vi "Run_Wavedump.vi"(6 "Close":bool, 7 "Start":bool, 8 "Channel":string[](array[string]), 9 "PMTs":string[](array[string]), 11 "Test":string(combo)) -> (0 "Error":string="\n", 1 "Event Build Error":bool, 2 "Over Temperature":bool, 3 "Command Line Output":string)   [LabVIEW 2018]
panel:
  in  "Tab Control":enum32{"Controls", "Read Me"}(tab)
  out "Files Moved":bool
  out "Bash Script Run":bool=TRUE
  in  "View PMT Files":bool
  in  "Run":string
  in  "Time":string
  # "This application is used to send a command to run the bash script relating to an electrical test for PMTs.\n\nThe bash script will run wavedump in a preset configuration.\n\nUse the Controls tab to send the necessary commands.\n\nTo run, enter up to 8 PMT numbers and the channels they are connected to on the digitiser.\n\nSelect the test to run and press \"Start\".\n\nA window will pop up to display the waveform as it is being recorded.\n\nTo view other PMT files or scroll through the ones being recorded, press \"View PMT Files\".\n\nAs the program only sends a command, it can't be used to stop or control wavedump.\n\nPress \"CLOSE\" to close the application."
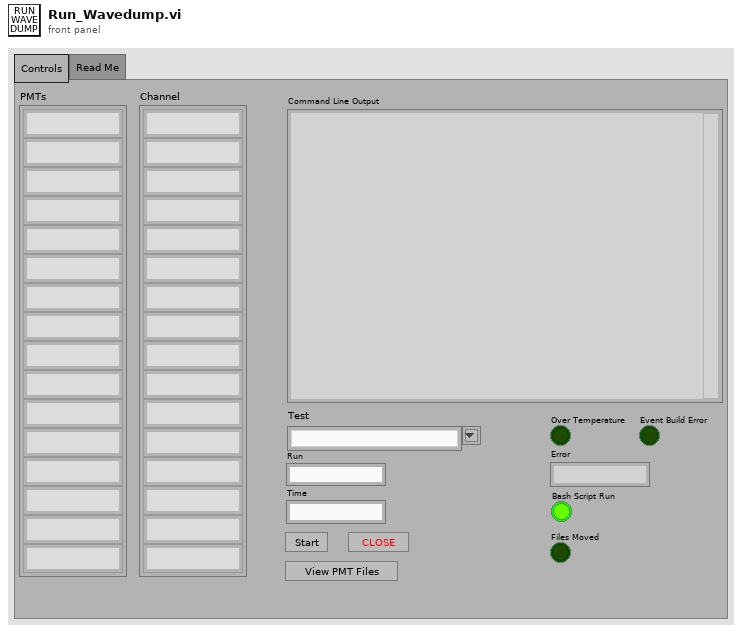
[diagram p1: front panel]
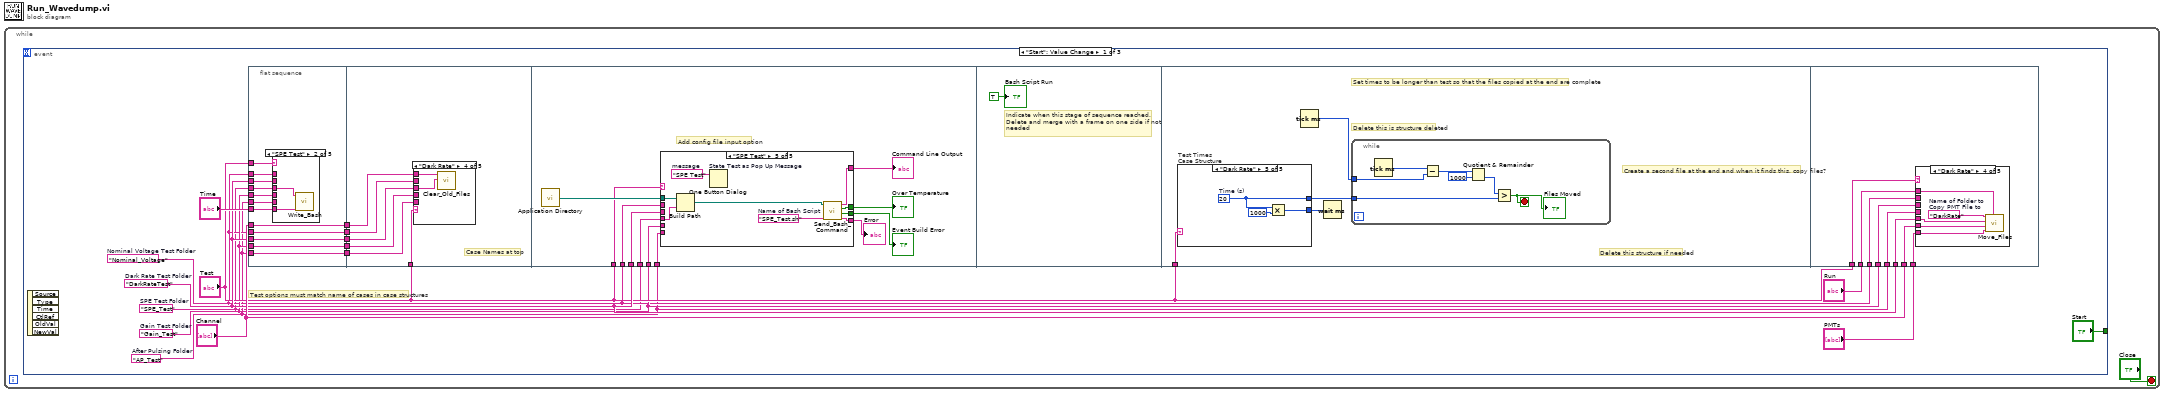
[diagram p0: block diagram]
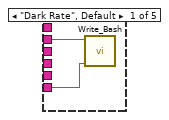
[diagram p2: hidden frame]
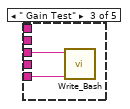
[diagram p3: hidden frame]
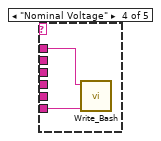
[diagram p4: hidden frame]
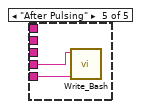
[diagram p5: hidden frame]
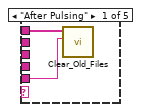
[diagram p6: hidden frame]
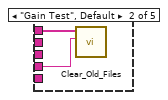
[diagram p7: hidden frame]
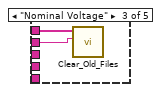
[diagram p8: hidden frame]
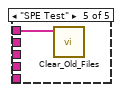
[diagram p9: hidden frame]
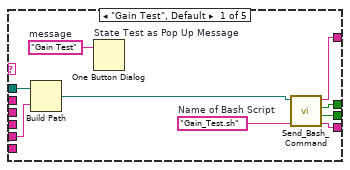
[diagram p10: hidden frame]
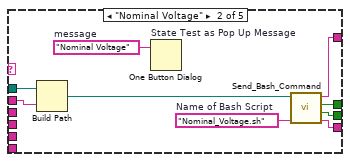
[diagram p11: hidden frame]
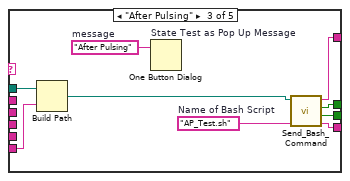
[diagram p12: hidden frame]
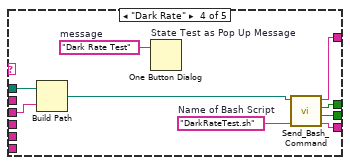
[diagram p13: hidden frame]
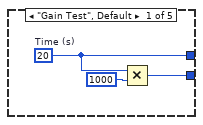
[diagram p14: hidden frame]
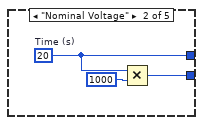
[diagram p15: hidden frame]
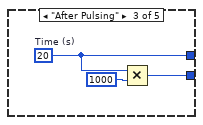
[diagram p16: hidden frame]
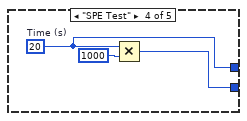
[diagram p17: hidden frame]
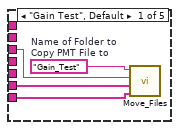
[diagram p18: hidden frame]
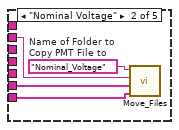
[diagram p19: hidden frame]
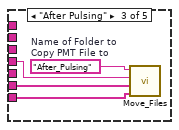
[diagram p20: hidden frame]
diagram:
  n1 = while {
    stop <- "Close" stop-if-true
    n2 = event shown="[0] \"Start\": Value Change" {
      selector: _ -> [_ _ _]
      dyn-events: _ -> [_ _ _]
      timeout: _ -> [_ _ _]
      tunnel: ["Start" "View PMT Files" w170] -> _
      event "Start": Value Change {
        w2 = "SPE_Test"  # SPE Test Folder
        w3 = "AP_Test"  # After Pulsing Folder
        w7 = "DarkRateTest"  # Dark Rate Test Folder
        w4 = "Nominal_Voltage"  # Nominal Voltage Test Folder
        w5 = "Gain_Test"  # Gain Test Folder
        # "Test options must match name of cases in case structures"
        n3 = event-data() -> ()  [unwired: 1 in, 6 out]
        n4 = flat-sequence {
          tunnel: w5 -> [w25]
          tunnel: w3 -> [w26]
          tunnel: w7 -> [w27]
          tunnel: w4 -> [w28]
          tunnel: "Channel" -> [w29]
          tunnel: [w29] -> w13
          tunnel: [w28] -> w12
          tunnel: [w27] -> w11
          tunnel: [w26] -> w10
          tunnel: [w25] -> w9
          tunnel: "Test" -> [w24]
          tunnel: "Time" -> [w23]
          tunnel: w7 -> [w22]
          tunnel: w5 -> [w21]
          tunnel: w4 -> [w20]
          tunnel: w3 -> [w19]
          tunnel: w2 -> [w18]
          tunnel: w13 -> [w45]
          tunnel: w12 -> [w44]
          tunnel: w11 -> [w43]
          tunnel: w10 -> [w42]
          tunnel: w9 -> [w41]
          tunnel: "Test" -> [w40]
          tunnel: "Test" -> [w60]
          tunnel: w5 -> [w59]
          tunnel: w4 -> [w58]
          tunnel: w7 -> [w57]
          tunnel: w3 -> [w56]
          tunnel: w2 -> [w55]
          tunnel: "Test" -> [w114]
          tunnel: "PMTs" -> [w142]
          tunnel: "Test" -> [w145]
          tunnel: w3 -> [w144]
          tunnel: "Channel" -> [w143]
          tunnel: w7 -> [w141]
          tunnel: w5 -> [w140]
          tunnel: w4 -> [w139]
          tunnel: "Run" -> [w138]
          frame #0 {
            n5 = case shown="\"SPE Test\"" w24 {
              tunnel: w23 -> [w31 w33 w34 w36 w38]
              tunnel: w22 -> [w30 _ _ _ _]
              tunnel: w21 -> [_ _ w35 _ _]
              tunnel: w20 -> [_ _ _ w37 _]
              tunnel: w19 -> [_ _ _ _ w39]
              tunnel: w18 -> [_ w32 _ _ _]
              frame "Dark Rate", Default {
                n6 = call "Write_Bash.vi"("Time"=w31, "Test"=w30) -> ()  [unwired: 10 in]
              }
              frame "SPE Test" {
                n7 = call "Write_Bash.vi"("Time"=w33, "Test"=w32) -> ()  [unwired: 10 in]
              }
              frame " Gain Test" {
                n8 = call "Write_Bash.vi"("Time"=w34, "Test"=w35) -> ()  [unwired: 10 in]
              }
              frame "Nominal Voltage" {
                n9 = call "Write_Bash.vi"("Time"=w36, "Test"=w37) -> ()  [unwired: 10 in]
              }
              frame "After Pulsing" {
                n10 = call "Write_Bash.vi"("Time"=w38, "Test"=w39) -> ()  [unwired: 10 in]
              }
            }
          }
          frame #1 {
            # "Case Names at top"
            n11 = case shown="\"Dark Rate\"" w40 {
              tunnel: w45 -> [w47 w49 w51 w53 w54]
              tunnel: w44 -> [_ _ w50 _ _]
              tunnel: w43 -> [_ _ _ w52 _]
              tunnel: w42 -> [w46 _ _ _ _]
              tunnel: w41 -> [_ w48 _ _ _]
              frame "After Pulsing" {
                n12 = call "Clear_Old_Files.vi"("Bash Script Folder Name"=w46, "Channel"=w47) -> ()  [unwired: 10 in]
              }
              frame "Gain Test", Default {
                n13 = call "Clear_Old_Files.vi"("Bash Script Folder Name"=w48, "Channel"=w49) -> ()  [unwired: 10 in]
              }
              frame "Nominal Voltage" {
                n14 = call "Clear_Old_Files.vi"("Bash Script Folder Name"=w50, "Channel"=w51) -> ()  [unwired: 10 in]
              }
              frame "Dark Rate" {
                n15 = call "Clear_Old_Files.vi"("Bash Script Folder Name"=w52, "Channel"=w53) -> ()  [unwired: 10 in]
              }
              frame "SPE Test" {
                n16 = call "Clear_Old_Files.vi"("Channel"=w54) -> ()  [unwired: 11 in]
              }
            }
          }
          frame #2 {
            # "Add config file input option"
            n17 = call <vilib>:"Application Directory.vi"() -> ("Application Directory"=w65:path)
            n18 = case shown="\"SPE Test\"" w60 {
              tunnel: [w66 w75 w84 w93 w103] -> w61
              tunnel: [w67 w76 w85 w94 w104] -> w62
              tunnel: [w68 w77 w86 w95 w105] -> w63
              tunnel: [w69 w78 w87 w96 w106] -> w64
              tunnel: w65 -> [w71 w80 w88 w99 w107]
              tunnel: w59 -> [w70 _ _ _ _]
              tunnel: w58 -> [_ w79 _ _ _]
              tunnel: w57 -> [_ _ _ w97 _]
              tunnel: w56 -> [_ _ w89 _ _]
              tunnel: w55 -> [_ _ _ _ w102]
              frame "Gain Test", Default {
                w73 = "Gain Test"  # message
                w74 = "Gain_Test.sh"  # Name of Bash Script
                n19 = Build Path(base path=w71, name or relative path=w70) -> (appended path=w72:path)
                n20 = One Button Dialog "State Test as Pop Up Message"(message=w73) -> ()  [unwired: 1 in, 1 out]
                n21 = call "Send_Bash_Command.vi"("working directory"=w72, "Bash script"=w74) -> ("Command Line Output"=w69:string, "Over Temperature"=w68:bool, "Event Build Error"=w67:bool, "Error"=w66:string)  [unwired: 5 in]
              }
              frame "Nominal Voltage" {
                w82 = "Nominal Voltage"  # message
                w83 = "Nominal_Voltage.sh"  # Name of Bash Script
                n22 = Build Path(base path=w80, name or relative path=w79) -> (appended path=w81:path)
                n23 = One Button Dialog "State Test as Pop Up Message"(message=w82) -> ()  [unwired: 1 in, 1 out]
                n24 = call "Send_Bash_Command.vi"("working directory"=w81, "Bash script"=w83) -> ("Command Line Output"=w78:string, "Over Temperature"=w77:bool, "Event Build Error"=w76:bool, "Error"=w75:string)  [unwired: 5 in]
              }
              frame "After Pulsing" {
                w91 = "After Pulsing"  # message
                w92 = "AP_Test.sh"  # Name of Bash Script
                n25 = Build Path(base path=w88, name or relative path=w89) -> (appended path=w90:path)
                n26 = One Button Dialog "State Test as Pop Up Message"(message=w91) -> ()  [unwired: 1 in, 1 out]
                n27 = call "Send_Bash_Command.vi"("working directory"=w90, "Bash script"=w92) -> ("Command Line Output"=w87:string, "Over Temperature"=w86:bool, "Event Build Error"=w85:bool, "Error"=w84:string)  [unwired: 5 in]
              }
              frame "Dark Rate" {
                w101 = "Dark Rate Test"  # message
                w98 = "DarkRateTest.sh"  # Name of Bash Script
                n28 = Build Path(base path=w99, name or relative path=w97) -> (appended path=w100:path)
                n29 = One Button Dialog "State Test as Pop Up Message"(message=w101) -> ()  [unwired: 1 in, 1 out]
                n30 = call "Send_Bash_Command.vi"("working directory"=w100, "Bash script"=w98) -> ("Command Line Output"=w96:string, "Over Temperature"=w95:bool, "Event Build Error"=w94:bool, "Error"=w93:string)  [unwired: 5 in]
              }
              frame "SPE Test" {
                w109 = "SPE Test"  # message
                w110 = "SPE_Test.sh"  # Name of Bash Script
                n31 = Build Path(base path=w107, name or relative path=w102) -> (appended path=w108:path)
                n32 = One Button Dialog "State Test as Pop Up Message"(message=w109) -> ()  [unwired: 1 in, 1 out]
                n33 = call "Send_Bash_Command.vi"("working directory"=w108, "Bash script"=w110) -> ("Command Line Output"=w106:string, "Over Temperature"=w105:bool, "Event Build Error"=w104:bool, "Error"=w103:string)  [unwired: 5 in]
              }
            }
            "Command Line Output" <- w64
            "Over Temperature" <- w63
            "Event Build Error" <- w62
            "Error" <- w61
          }
          frame #3 {
            # "Indicate when this stage of sequence reached.\nDelete and merge with a frame on one side if not needed"
            "Bash Script Run" <- TRUE
          }
          frame #4 {
            # "Create a second file at the end and when it finds this, copy files?"
            # "Delete this is structure deleted"
            # "Delete this structure if needed"
            # "Set times to be longer than test so that the files copied at the end are complete"
            n34 = case "Test Times\nCase Structure" shown="\"Dark Rate\"" w114 {
              tunnel: [w124 w127 w130 w133 w137] -> w115
              tunnel: [w123 w126 w129 w132 w135] -> w112
              frame "Gain Test", Default {
                w123 = u32 20  # Time (s)
                n35 = Multiply(x=w123, y=u32 1000) -> (x*y=w124:u32)
              }
              frame "Nominal Voltage" {
                w126 = u32 20  # Time (s)
                n36 = Multiply(x=w126, y=u32 1000) -> (x*y=w127:u32)
              }
              frame "After Pulsing" {
                w129 = u32 20  # Time (s)
                n37 = Multiply(x=w129, y=u32 1000) -> (x*y=w130:u32)
              }
              frame "SPE Test" {
                w132 = u32 20  # Time (s)
                n38 = Multiply(x=w132, y=u32 1000) -> (x*y=w133:u32)
              }
              frame "Dark Rate" {
                w135 = u32 20  # Time (s)
                n39 = Multiply(x=w135, y=u32 1000) -> (x*y=w137:u32)
              }
            }
            n40 = Tick Count (ms)() -> (millisecond timer value=w113:u32)
            n41 = Wait (ms)(milliseconds to wait=w115) -> ()  [unwired: 1 out]
            n42 = while {
              tunnel: w113 -> [w121]
              tunnel: w112 -> [w117]
              stop <- w116 stop-if-true
              n43 = Tick Count (ms)() -> (millisecond timer value=w122:u32)
              n44 = Subtract(x=w122, y=w121) -> (x-y=w120:u32)
              n45 = Quotient & Remainder(x=w120, y=u32 1000) -> (floor(x/y)=w118:u32)  [unwired: 1 out]
              n46 = Greater?(x=w118, y=w117) -> (0:w116:bool)
              "Files Moved" <- w116
            }
          }
          frame #5 {
            n47 = case shown="\"Dark Rate\"" w145 {
              tunnel: w144 -> [_ _ w157 _ _]
              tunnel: w143 -> [w147 w151 w155 w160 w164]
              tunnel: w142 -> [w146 w150 w154 w159 w163]
              tunnel: w141 -> [_ _ _ w161 _]
              tunnel: w140 -> [w148 _ _ _ _]
              tunnel: w139 -> [_ w152 _ _ _]
              tunnel: w138 -> [_ _ _ w158 _]
              frame "Gain Test", Default {
                w149 = "Gain_Test"  # Name of Folder to Copy PMT File to
                n48 = call "Move_Files.vi"("PMTs"=w146, "Channel"=w147, "Folder Containing Bash Script"=w148, "Name of Folder to\nCopy PMT File to"=w149) -> ()  [unwired: 8 in]
              }
              frame "Nominal Voltage" {
                w153 = "Nominal_Voltage"  # Name of Folder to Copy PMT File to
                n49 = call "Move_Files.vi"("PMTs"=w150, "Channel"=w151, "Folder Containing Bash Script"=w152, "Name of Folder to\nCopy PMT File to"=w153) -> ()  [unwired: 8 in]
              }
              frame "After Pulsing" {
                w156 = "After_Pulsing"  # Name of Folder to Copy PMT File to
                n50 = call "Move_Files.vi"("PMTs"=w154, "Channel"=w155, "Folder Containing Bash Script"=w157, "Name of Folder to\nCopy PMT File to"=w156) -> ()  [unwired: 8 in]
              }
              frame "Dark Rate" {
                w162 = "DarkRate"  # Name of Folder to Copy PMT File to
                n51 = call "Move_Files.vi"("Run"=w158, "PMTs"=w159, "Channel"=w160, "Folder Containing Bash Script"=w161, "Name of Folder to\nCopy PMT File to"=w162) -> ()  [unwired: 7 in]
              }
              frame "SPE Test" {
                w165 = "SPE_Test"  # Name of Folder to Copy PMT File to
                n52 = call "Move_Files.vi"("PMTs"=w163, "Channel"=w164, "Name of Folder to\nCopy PMT File to"=w165) -> ()  [unwired: 9 in]
              }
            }
          }
        }
      }
      event "View PMT Files": Value Change {
        n53 = event-data() -> ()  [unwired: 1 in, 6 out]
        n54 = call <vilib>:"Application Directory.vi"() -> ("Application Directory"=w166:path)
        n55 = call <vilib>:"System Exec.vi"("working directory"=w166, "command line"="./ReadPMTFiles") -> ()  [unwired: 6 in, 4 out]
      }
      event "Close": Value Change {
        n56 = event-data() -> ("NewVal"=w170:bool)  [unwired: 1 in, 5 out]
        n57 = control-ref of="This VI"() -> (w169:refnum<vi>)
        n58 = invoke class="VI" method="FP.Close"(reference=w169) -> ()  [unwired: 2 in, 3 out]
      }
    }
  }
